vi "Word class path.vi"() -> (8 "Word class path":path)   [LabVIEW 2017, in "NI_ReportGenerationCore.lvlib"]
uses:
  <vilib>/Utility/NIReport.llb/NI_ReportGenerationCore.lvlib
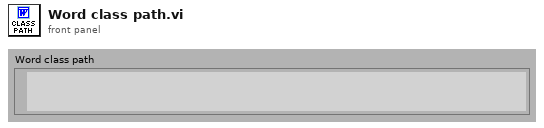
[diagram p1: front panel]
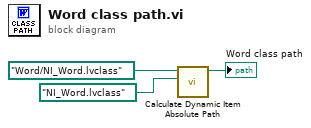
[diagram p0: block diagram]
diagram:
  n1 = call <vilib>:"Calculate Dynamic Item Absolute Path.vi"("Compat Built App Relative Path"=path "NI_Word.lvclass" ("path"), "Core Relative Path"=path "Word/NI_Word.lvclass" ("path")) -> ("Resulting Absolute Path"=→"Word class path":path)  [unwired: 9 out]
